vi "Control_Freeze.vi"(3 "에러 입력(에러 없음)":errorcluster, 4 "Timeout (ms)":i32, 5 "TCP 네트워크 연결 입력":refnum<k5>) -> (0 "에러 출력":errorcluster, 2 "TCP 네트워크 연결 출력":refnum<k5>)   [LabVIEW 2016]
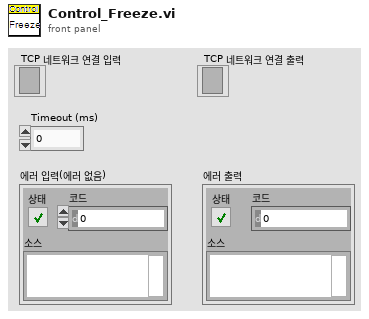
[diagram p1: front panel]
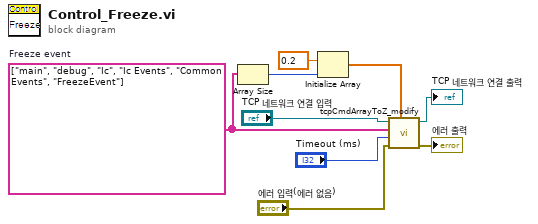
[diagram p0: block diagram]
diagram:
  w3 = string[] ["main", "debug", "Ic", "Ic Events", "Common Events", "FreezeEvent"]  # Freeze event
  n1 = Array Size(array=w3) -> (size(s)=w1:i32)
  n2 = Initialize Array(0.2 ("element"), w1) -> (w4:dbl[])
  n3 = call "tcpCmdArrayToZ_modify.vi"("Delay (sec)"=w4, "error in (no error)"="에러 입력(에러 없음)", "Timeout (ms)"="Timeout (ms)", "Command array"=w3, "connection ID in"="TCP 네트워크 연결 입력") -> ("error out"=→"에러 출력":errorcluster, "connection ID out"=→"TCP 네트워크 연결 출력":refnum<k5>)  [unwired: 2 in, 3 out]
